vi "Queue init.vi"(10 "Message Cluster":T1, 11 "name (unnamed)":string) -> (3 "Cluster":T2)   [LabVIEW 2015]
uses:
  QMH Fundamentals - Message Cluster.ctl
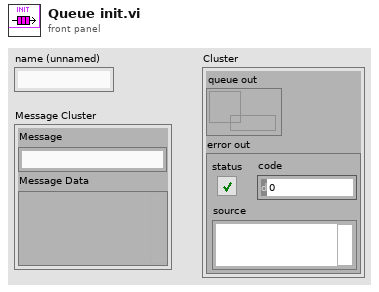
[diagram p1: front panel]
types:
  T1 = typedef "QMH Fundamentals - Message Cluster.ctl" = cluster{"Message":string, "Message Data":variant}
  T2 = cluster{"queue out":refnum<queue>, "error out":errorcluster}
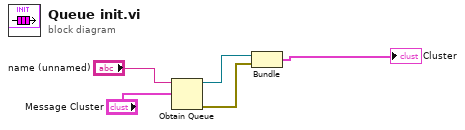
[diagram p0: block diagram]
diagram:
  n1 = Obtain Queue(name (unnamed)="name (unnamed)", element data type="Message Cluster") -> (queue out=w2:refnum<queue>, error out=w3:errorcluster)  [unwired: 3 in, 1 out]
  n2 = Bundle("queue out"=w2, "error out"=w3) -> (→"Cluster":T2)  [unwired: 1 in]
